vi "Stopping.vi"(6 "Teller":T1 {"Time" format="%<%x %.3X>T"}, 8 "Error in":errorcluster, 11 "TEMPLATE Actor in":refnum<class "TEMPLATE Actor.lvclass">) -> (0 "Error out":errorcluster, 3 "TEMPLATE Actor out":refnum<class "TEMPLATE Actor.lvclass">)   [LabVIEW 2020, in "_Template.lvlib" / "Templates.lvlib" / "TEMPLATE jettl Actor.lvlib" / "TEMPLATE Actor.lvlib" / "TEMPLATE Actor.lvclass"]
doc: "jettl 6.12.1.94\nNathan Davis - Nathan Davis\nCopyright (c) 2026, Nathan Davis\nMIT"
uses:
  TEMPLATE Actor.lvclass
  TEMPLATE Actor.lvclass/TEMPLATE Actor.ctl
  C:/git/jettl/src/jettl Tools/_Template/Templates/TEMPLATE jettl Actor/TEMPLATE Actor/TEMPLATE Actor/TEMPLATE Actor.lvclass
  C:/git/jettl/src/jettl/jettl/Actor/Actor.lvclass
  C:/git/jettl/src/jettl/jettl/Start jettl Msg/Start jettl Msg/Start jettl Msg.lvclass
  C:/git/jettl/src/jettl/jettl/Stop jettl Msg/Stop jettl Msg/Stop jettl Msg.lvclass
  C:/git/jettl/src/jettl/jettl/Stopped jettl Msg/Stopped jettl Msg/Stopped jettl Msg.lvclass
  C:/git/jettl/src/jettl/jettl/Stopping jettl Msg/Stopping jettl Msg/Stopping jettl Msg.lvclass
  jettl/jettl/Stopping jettl Msg/Stopping/Stopping.lvlib
  jettl/jettl/Stopping jettl Msg/Stopping/Recurse.vi
  jettl/jettl/Relation.ctl
  jettl/jettl/jettl.lvlib
  jettl/jettl/Teller Metadata/Teller Metadata.lvclass
  jettl/jettl/Teller.ctl
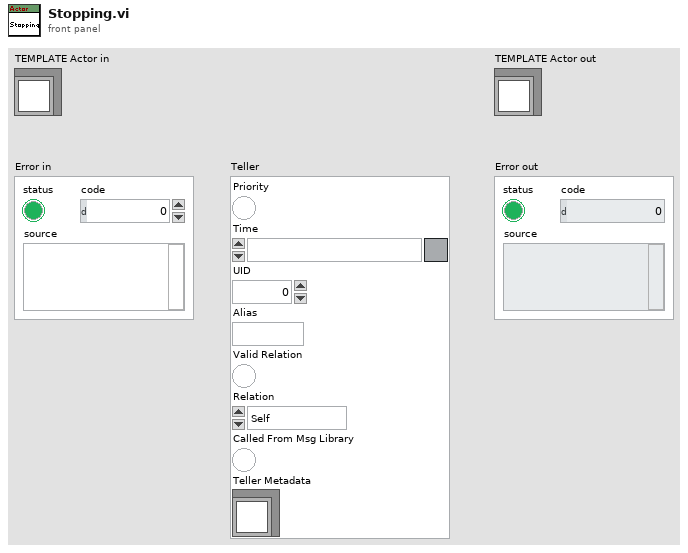
[diagram p1: front panel]
types:
  T1 = typedef "jettl.lvlib/Teller.ctl" = cluster{"Priority":bool, "Time":timestamp, "UID":i32, "Alias":string, "Valid Relation":bool, "Relation":T2, "Called From Msg Library":bool, "Teller Metadata":refnum<class "Teller Metadata.lvclass">}
  T2 = typedef "jettl.lvlib/Relation.ctl" = enum16{"Self", "Parent", "Child"}
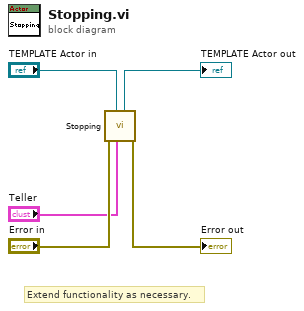
[diagram p0: block diagram]
diagram:
  # "Extend functionality as necessary."
  n1 = call-poly "Stopping.vi"("Teller"="Teller", "Actor in"="TEMPLATE Actor in", "Error in"="Error in") -> ("Error out"=→"Error out":errorcluster, "Actor out"=→"TEMPLATE Actor out":refnum<class "TEMPLATE Actor.lvclass">)  [unwired: 7 in]
